vi "Results to Waveforms (array of timestamps).vi"(1 "data type":timestamp[][](array[timestamp]), 7 "result references":T1[](array[typedef]), 11 "error in (no error)":errorcluster) -> (6 "signals out":timestamp[][](array[timestamp]), 8 "result references out":T1[](array[typedef]), 15 "error out":errorcluster)   [LabVIEW 2020, in "NI_DataFinder.lvlib"]
doc: "Extracts the signals from the results of a DataFinder search."
uses:
  <vilib>/DataFinder/NI_DataFinder.lvlib
  <vilib>/userdefined/DFSearchResult.ctl
  <vilib>/userdefined/NI_DataFinder Controls.lvlib
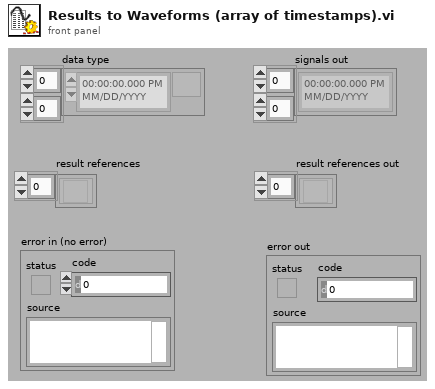
[diagram p1: front panel]
types:
  T1 = typedef "NI_DataFinder Controls.lvlib/DFSearchResult.ctl" = refnum<k20>
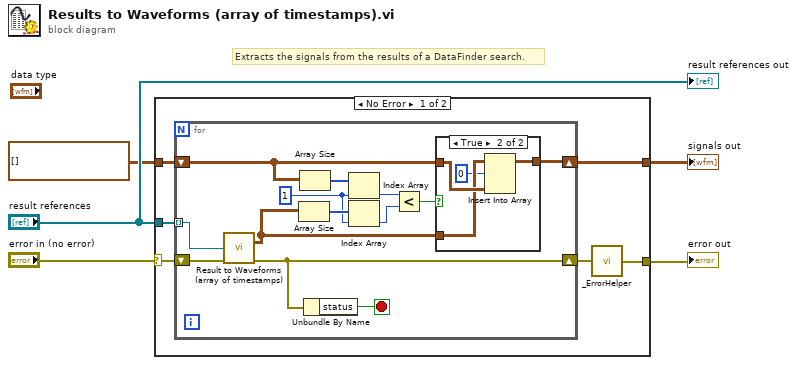
[diagram p0: block diagram]
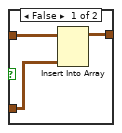
[diagram p2: hidden frame]
diagram:
  # "Extracts the signals from the results of a DataFinder search."
  n1 = case shown="No Error" "error in (no error)" {
    selector: "error in (no error)" -> [w6 w32]
    tunnel: "result references" -> [w11 _]
    tunnel: timestamp[][] [] ("signals out") -> [w10 w33]
    tunnel: [w9 w32] -> w3
    tunnel: [w7 w33] -> w2
    frame No Error {
      n2 = for {
        shift-right: [w14] -> w7
        shift-left: w10 -> [w13]
        tunnel: w11 -> [w24] mode=indexing
        shift-right: [w21] -> w8
        shift-left: w6 -> [w23]
        stop <- w22 stop-if-true
        w18 = 1 ("index")
        n3 = call <vilib>:"Result to Waveforms (array of timestamps).vi"("result reference"=w24, "error in"=w23) -> ("signals out"=w12:timestamp[][], "error out"=w21:errorcluster)  [unwired: 2 in, 10 out]
        n4 = Array Size(array=w12) -> (size(s)=w19:i32[])
        n5 = Array Size(array=w13) -> (size(s)=w20:i32[])
        n6 = Unbundle By Name(w21) -> ("status"=w22:bool)
        n7 = Index Array(array=w20, index=w18) -> (element=w16:i32)
        n8 = Index Array(array=w19, index=w18) -> (element=w17:i32)
        n9 = Less?(x=w16, y=w17) -> (x < y?=w15:bool)
        n10 = case shown="True" w15 {
          tunnel: w13 -> [w26 w31]
          tunnel: w12 -> [w27 w30]
          tunnel: [w25 w28] -> w14
          frame False {
            n11 = Insert Into Array(array=w26, new element=w27) -> (w25:timestamp[][])  [unwired: 2 in]
          }
          frame True {
            n12 = Insert Into Array(array=w30, index (row)=0, new element=w31) -> (w28:timestamp[][])  [unwired: 1 in]
          }
        }
      }
      n13 = call <vilib>:"_ErrorHelper.vi"("error IO"=w8) -> ("error out"=w9:errorcluster)
    }
    frame Error {
    }
  }
  "error out" <- w3
  "signals out" <- w2
  "result references out" <- "result references"
